vi "Door-Close.vi"(7 "Door reference":refnum<vi>, 8 "error in (no error)":errorcluster, 9 "Eventstring":string="auto-generate") -> (0 "error out":errorcluster)   [LabVIEW 2015]
doc: "Closes a door.\n\nDoor reference: which door to close?\nEventstring: used for timestamping\n--empty: no timestamp will be generated\n--unwired or \"auto-generate\": TS w/ default eventstring\n--otherwise: TS with user-provided string\n\nThe default eventstring is:\n[door name].close\nwhere [door name] is the referenced door's front panel label text."
uses:
  Typedefs/Door.ctl
  Rack/Typedefs/OutputRequest refnum.ctl
  Rack/Typedefs/OutputRequest.ctl
  Rack/Typedefs/InputData cluster.ctl
  Rack/Methods/Port drivers/DigitalInput-DataCluster.ctl
panel:
  # "Duration"
  # "Active hi?"
  # "Open"
  # "Close"
  # "(must be on the same \ndevice as open/close)"
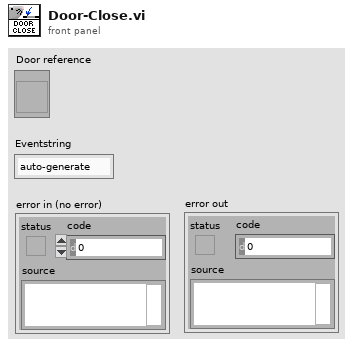
[diagram p1: front panel]
types:
  T1 = typedef "Door.ctl" = cluster{"Open":bool, "Settings":cluster{"Open active hi?":bool, "Open duration":i32, "Close duration":i32, "Close active hi?":bool, "Open portname":string, "Open idx":i32, "Close portname":string, "Close idx":i32, "Timestamp portname":string}, "OutputRequest event ref":T2, "InputData reference":refnum<vi>}
  T2 = typedef "OutputRequest refnum.ctl" = refnum<user-event>
  T3 = typedef "OutputRequest.ctl" = cluster{"Target":string, "Command":string}
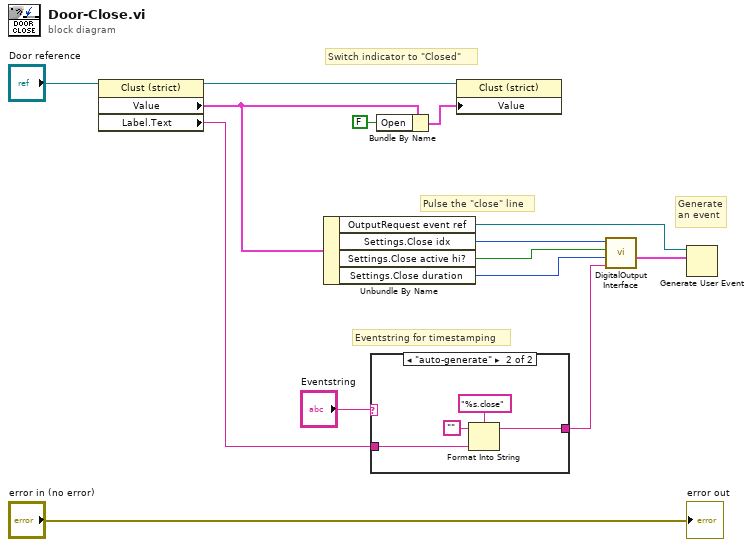
[diagram p0: block diagram]
diagram:
  # "Switch indicator to \"Closed\""
  # "Eventstring for timestamping"
  # "Generate\nan event"
  # "Pulse the \"close\" line"
  n1 = property class="Clust (strict)"(reference="Door reference") -> (reference out=w6:refnum<vi>, "Value"=w5:T1, "Label.Text"=w11:string)  [unwired: 1 in, 1 out]
  n2 = Unbundle By Name(w5) -> ("OutputRequest event ref"=w1:T2, "Settings.Close idx"=w13:i32, "Settings.Close active hi?"=w8:bool, "Settings.Close duration"=w7:i32)
  n3 = case shown="\"auto-generate\"" "Eventstring" {
    selector: "Eventstring" -> [w15 _]
    tunnel: w11 -> [_ w17]
    tunnel: [w15 w16] -> w10
    frame Default {
      # "Use user-provided string"
    }
    frame "auto-generate" {
      n4 = Format Into String(format string="%s.close", initial string="", w17) -> (resulting string=w16:string)  [unwired: 1 in, 1 out]
    }
  }
  n5 = Bundle By Name(cluster=w5, "Open"=FALSE) -> (w4:T1)
  n6 = property class="Clust (strict)"(reference=w6, "Value"=w4) -> ()  [unwired: 1 in, 2 out]
  n7 = call "DigitalOutput Interface.vi"("Eventstring"=w10, "Pulse duration (-1 for cont.)"=w7, "On/off"=w8, "Port index"=w13) -> ("OutputRequest"=w9:T3)  [unwired: 7 in]
  n8 = Generate User Event(user event=w1, event data cluster=w9) -> ()  [unwired: 2 in, 2 out]
  "error out" <- "error in (no error)"
